vi "velleman-init.vi"(5 "Shutter VIS":bool, 6 "Shutter UV":bool, 7 "Power Control":bool) -> (0 "isActive":bool, 1 "Shutter UV 2":bool, 2 "Shutter VIS 2":bool, 3 "Power Control 2":bool)   [LabVIEW 2015]
uses:
  other/velleman/K8055D.dll
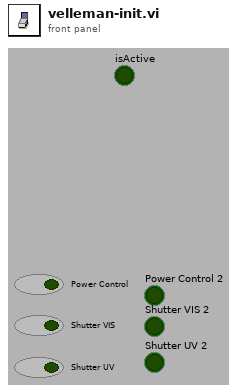
[diagram p1: front panel]
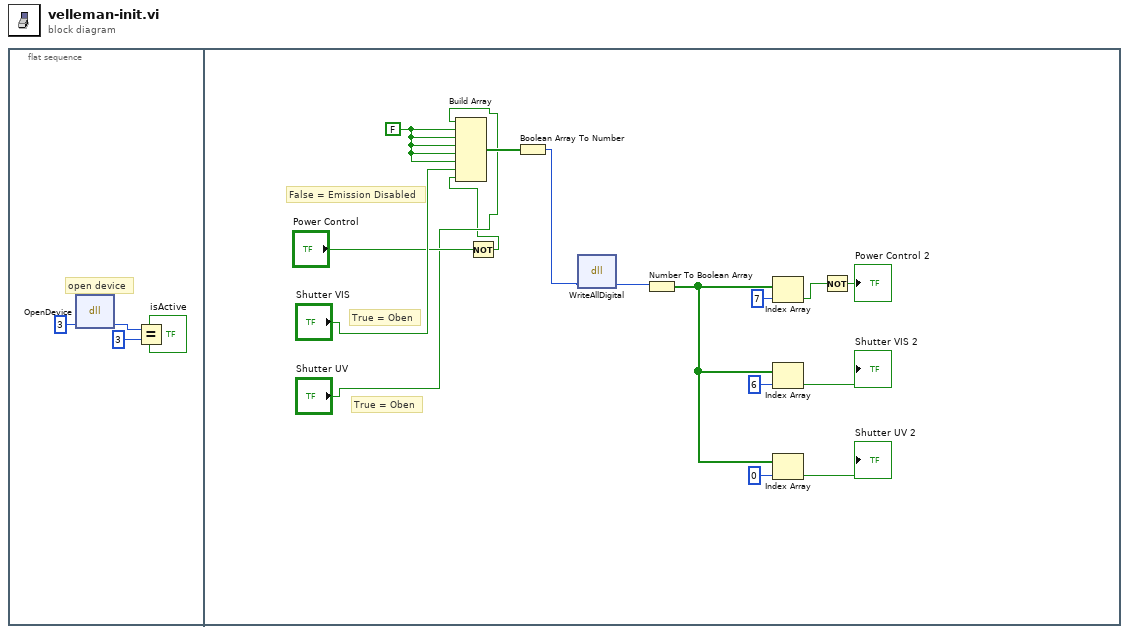
[diagram p0: block diagram]
diagram:
  n1 = flat-sequence {
    frame #0 {
      # "open device"
      n2 = dll-call lib="D:/Programs/LabView/playground/PLEMv3/other/velleman/K8055D.dll" fn="OpenDevice"(3) -> (w3:i32)  [unwired: 4 in, 2 out]
      n3 = Equal?(x=w3, y=3) -> (x = y?=→"isActive":bool)
    }
    frame #1 {
      w20 = FALSE
      # "True = Oben"
      # "False = Emission Disabled"
      # "True = Oben"
      n4 = Not(x="Power Control") -> (.not. x?=w5:bool)
      n5 = Build Array("Shutter UV", w20, w20, w20, w20, w20, "Shutter VIS", w5) -> (w19:bool[])
      n6 = Boolean Array To Number(Boolean array=w19) -> (number=w17:u32)
      n7 = dll-call lib="D:/Programs/LabView/playground/PLEMv3/other/velleman/K8055D.dll" fn="WriteAllDigital"(w17) -> (w16:i32)  [unwired: 4 in, 2 out]
      n8 = Number To Boolean Array(number=w16) -> (Boolean array=w10:bool[])
      n9 = Index Array(array=w10, index=7) -> (element=w7:bool)
      n10 = Index Array(array=w10, index=6) -> (element=→"Shutter VIS 2":bool)
      n11 = Index Array(array=w10, index=0) -> (element=→"Shutter UV 2":bool)
      n12 = Not(x=w7) -> (.not. x?=→"Power Control 2":bool)
    }
  }
